vi "Add Compare to List.vi"(8 "error in (no error)":errorcluster, 9 "Bit type":T1, 11 "I2C waveform info":T2) -> (0 "error out":errorcluster, 3 "I2C waveform info out":T2)   [LabVIEW 2009, in "IDW.lvlib"]
doc: "Adds the current sample offset (contained in the <b>I2C waveform info</b> cluster) to the list of compare locations and adds the <b>Bit type</b> to the list of compare types."
uses:
  IDW.lvlib
  _Typedefs/Waveform info.ctl
  _Typedefs/Timing - ticks.ctl
  _Typedefs/Default transition action.ctl
  _Typedefs/Bit type.ctl
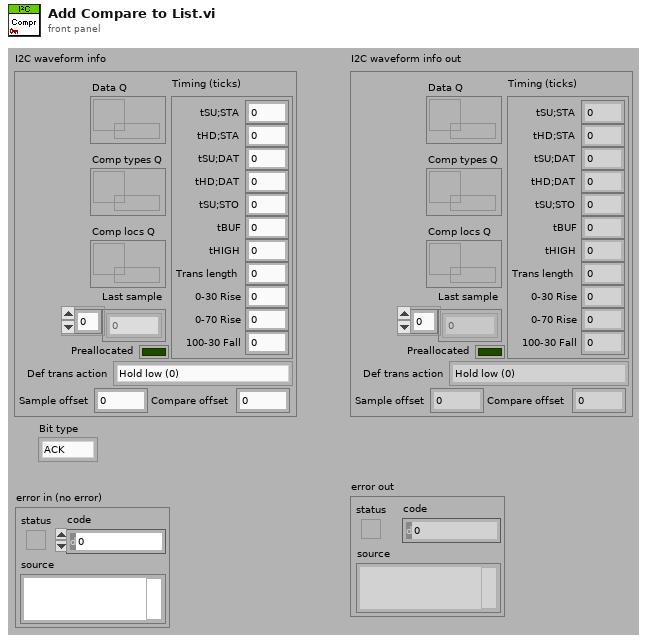
[diagram p1: front panel]
types:
  T1 = typedef "IDW.lvlib/Bit type.ctl" = enum16{"ACK", "Data"}
  T2 = typedef "IDW.lvlib/Waveform info.ctl" = cluster{"Last sample":u8[], "Sample offset":u64, "Compare offset":u64, "Timing (ticks)":T3, "Preallocated":bool, "Def trans action":T4, "Data Q":refnum<queue>, "Comp types Q":refnum<queue>, "Comp locs Q":refnum<queue>}
  T3 = typedef "IDW.lvlib/Timing - ticks.ctl" = cluster{"tSU;STA":i32, "tHD;STA":i32, "tSU;DAT":i32, "tHD;DAT":i32, "tSU;STO":i32, "tBUF":i32, "tHIGH":i32, "Trans length":i32, "0-30 Rise":i32, "0-70 Rise":i32, "100-30 Fall":i32}
  T4 = typedef "IDW.lvlib/Default transition action.ctl" = enum16{"Hold low (0)", "Release (Z)", "Set up next value", "Hold previous value", "Preserve tHD;DAT and tSU;DAT"}
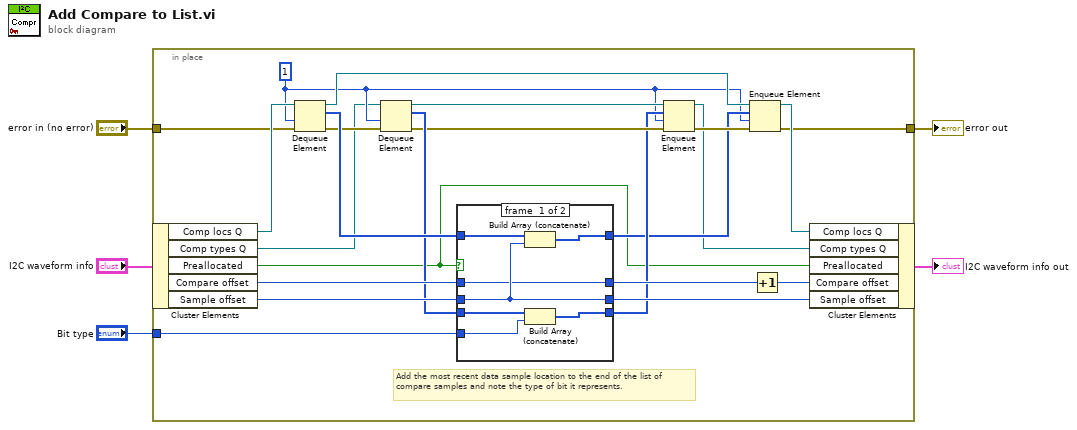
[diagram p0: block diagram]
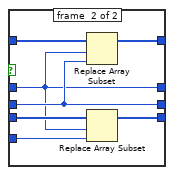
[diagram p2: hidden frame]
diagram:
  n1 = in-place {
    in-place-border: "Bit type" -> [w25]
    in-place-border: "error in (no error)" -> [w10]
    in-place-border: [w9] -> w1
    w11 = 1 ("timeout in ms (-1)")
    # "Add the most recent data sample location to the end of the list of compare samples and note the type of bit it represents."
    n2 = in-place-cluster #1("I2C waveform info") -> ("Comp locs Q"=w22:refnum<queue>, "Comp types Q"=w8:refnum<queue>, "Preallocated"=w6:bool, "Compare offset"=w26:u64, "Sample offset"=w28:u64)
    n3 = Dequeue Element(queue=w22, timeout in ms (-1)=w11, error in (no error)=w10) -> (queue out=w20:refnum<queue>, element=w19:u64[], error out=w17:errorcluster)  [unwired: 1 out]
    n4 = Dequeue Element(queue=w8, timeout in ms (-1)=w11, error in (no error)=w17) -> (queue out=w21:refnum<queue>, element=w18:T1[], error out=w16:errorcluster)  [unwired: 1 out]
    n5 = case shown="True" w6 {
      tunnel: w19 -> [w35 w42]
      tunnel: [w34 w41] -> w13
      tunnel: w28 -> [w33 w37]
      tunnel: w18 -> [w31 w40]
      tunnel: [w30 w39] -> w14
      tunnel: w26 -> [w32 w36]
      tunnel: w25 -> [w29 w38]
      tunnel: [w33 w37] -> w24
      tunnel: [w32 w36] -> w23
      frame #0 {
        n6 = Build Array (concatenate)(w35, w33) -> (w34:u64[])
        n7 = Build Array (concatenate)(w31, w29) -> (w30:T1[])
      }
      frame #1 {
        n8 = Replace Array Subset(array=w42, new element=w37, index=w36) -> (w41:u64[])
        n9 = Replace Array Subset(array=w40, new element=w38, index=w36) -> (w39:T1[])
      }
    }
    n10 = Enqueue Element(queue=w21, element=w14, timeout in ms (-1)=w11, error in (no error)=w16) -> (queue out=w7:refnum<queue>, error out=w15:errorcluster)  [unwired: 1 out]
    n11 = Enqueue Element(queue=w20, element=w13, timeout in ms (-1)=w11, error in (no error)=w15) -> (queue out=w12:refnum<queue>, error out=w9:errorcluster)  [unwired: 1 out]
    n12 = Increment(x=w23) -> (x+1=w27:u64)
    n13 = in-place-cluster #1("Comp locs Q"=w12, "Comp types Q"=w7, "Preallocated"=w6, "Compare offset"=w27, "Sample offset"=w24) -> (→"I2C waveform info out":T2)
  }
  "error out" <- w1
